vi "APC_9056_TS_loop.vi"(1 "DAQqueue":T3={"Queue array"=[0.0, 0.0, 0.0, 0.0, 0.0, 0.0, 0.0, 0.0, 0.0, 0.0, 0.0, 0.0, 0.0, 0.0, 0.0, 0.0, 0.0, 0.0, 0.0, 0.0, 0.0, 0.0, 0.0, 0.0, 0.0, 0.0, 0.0, 0.0, 0.0, 0.0, 0.0, 0.0, 0.0, 0.0, 0.0, 0.0, 0.0, 0.0, 0.0, 0.0, 0.0, 0.0, 0.0, 0.0, 0.0, 0.0, 0.0, 0.0, 0.0, 0.0, 0.0, 0.0, 0.0, 0.0, 0.0, 0.0, 0.0, 0.0, 0.0, 0.0, 0.0, 0.0, 0.0, 0.0, 0.0, 0.0, 0.0, 0.0, 0.0, 0.0, 0.0], "Channel list"=["TimeStamp9056", "NI9220_0_0", "NI9220_0_1", "NI9220_0_2", "NI9220_0_3", "NI9220_0_4", "NI9220_0_5", "NI9220_0_6", "NI9220_0_7", "NI9220_0_8", "NI9220_0_9", "NI9220_0_10", "NI9220_0_11", "NI9220_0_12", "NI9220_0_13", "NI9220_0_14", "NI9220_0_15", "NI9220_1_0", "NI9220_1_1", "NI9220_1_2", "NI9220_1_3", "NI9220_1_4", "NI9220_1_5", "NI9220_1_6", "NI9220_1_7", "NI9220_1_8", "NI9220_1_9", "NI9220_1_10", "NI9220_1_11", "NI9220_1_12", "NI9220_1_13", "NI9220_1_14", "NI9220_1_15", "Pcyl1", "Pcyl2", "Pcyl3", "Pcyl4", "time_9049_TS", "SystemState", "InjEnable", "MainEnable", "MainDuration", "MainSOI", "SparkEnable", "SparkTiming", "EngineSpeed_rpm", "SystPres", "IMEPg1", "IMEPg2", "IMEPg3", "IMEPg4", "IMEPg5", "IMEPg6", "IMEPn1", "IMEPn2", "IMEPn3", "IMEPn4", "IMEPn5", "IMEPn6", "MaxPcyl1", "MaxPcyl2", "MaxPcyl3", "MaxPcyl4", "MaxPcyl5", "MaxPcyl6", "IMEPstd1", "IMEPstd2", "IMEPstd3", "IMEPstd4", "IMEPstd5", "IMEPstd6"], "TS queue"=refnum, "TS signals path"="/home/lvuser/natinst/LabVIEW Data/APC_10Hz_"}, 2 "error in":errorcluster, 3 "scaled dAQmx task":refnum<k21>[](array[refnum])=["", "", ""]) -> ()   [LabVIEW 2020]
doc: "This example demonstrates the procedure required to apply different NI-DAQmx Custom Scales to each virtual channel in a task. A DAQmx Task Property Node (Functions >> NI Measurements >> DAQmx - Data Acquisition >> DAQmx Advanced Task Options) is used to obtain the task's virtual channels. A DAQmx Channel Property Node (Functions >> NI Measurements >> DAQmx - Data Acquisition) is then used to set the custom scale for each virtual channel in the task.\n\nThe \"DAQmx Create Scale\" VI creates a custom scale for each channel in the channel list. *Note, make sure your Minimum and Maximum channel parameters are consistent with the range the scale will create."
uses:
  controls/APC_ControlSettings.ctl
  controls/APC_PIDcontrolSettings.ctl
  <vilib>/Platform/TimedLoop/XDataNode/timing_clust.ctl
  <vilib>/Platform/TimedLoop/XDataNode/nitl_modes.ctl
  <vilib>/Platform/TimedLoop/XDataNode/wakeup.ctl
  <vilib>/DAQmx/read.llb/DAQmx Read (Analog 2D DBL NChan NSamp).vi
  <vilib>/Analysis/baseanly.llb/Mean (DBL).vi
  <vilib>/DAQmx/miscellaneous.llb/DAQmx Fill In Error Info.vi
  <vilib>/FPGAPlugInAG/cRIO-9056/niLvFpga_Open_cRIO-9056.vi
  <vilib>/rvi/interface/common/dynamic/niFpgaDynamicAddResources.vi
  <vilib>/Utility/error.llb/Error Cluster From Error Code.vi
  <vilib>/rvi/errors/niLvFpgaAdjustHostInterfaceError.vi
  <vilib>/Platform/TimedLoop/XDataNode/XDataNode.xnode
  <vilib>/rvi/interface/nirviOpenFPGA/nirviOpenFPGA.xnode
  FPGA Bitfiles/monarch_FPGATarget2_APC9056FPGAmain_1JKoecJL0LU.lvbitx
  APC_9056_FPGA_main.vi
  <vilib>/rvi/interface/nirviReadWriteControl/nirviReadWriteControl.xnode
  <vilib>/Platform/TimedLoop/XDataNode/XDNodeRunTimeDep.lvlib
  <vilib>/Analysis/NI_AALBase.lvlib
  <resource>/objmgr/daqmx.rc
  NiFpgaLv.dll
  <vilib>/rvi/interface/Simulation/niFpgaSimulationCallBeginRW.vi
  FPGA Bitfiles/monarch_FPGATarget3_APC9053FPGAmain_w2oHWSMkDKM.lvbitx
  APC_9053_FPGA_main.vi
panel:
  out "error out TEST":errorcluster
  out "task out_TEST":refnum<k21>
  out "NumChans_TEST":u32
  out "s? t:f":i8
  out "MTRnotResponding":bool
  out "PCnotResponding":bool
  out "9049notResponding":bool
  out "9056notResponding":bool
  out "PC_ControlSettings":T1={"Spark advance [CADBTDC]"=0.0, "Pref"=0.0, "O2ref"=0.0, "DI advance [CADBTDC]"=0.0, "DI duration [ms] "=0.0, "CO2ref"=0.0, "PFI duration [ms]"=0.0, "IMEP ref"=0.0, "Speed ref"=0.0, "IGN enable"=TRUE, "DI enable"=TRUE, "CL PFI\n lambda"=TRUE, "CL PFI\nIMEP"=FALSE, "Activate\ncylinder"=[FALSE, FALSE, FALSE, FALSE, FALSE, FALSE], "Force idling"=FALSE, "Force motoring"=FALSE, "ETP resync"=FALSE, "Requested mode"=0, "Clear Sync Errors"=FALSE, "toggle TDC"=FALSE, "l ref"=0.0, "PID control references"={"NG"=FALSE, "Ar"=FALSE, "O2"=FALSE, "Intake vent"=FALSE, "Cross vent"=FALSE, "Exhaust vent"=FALSE, "NG control mode"=0, "NG-FC-001-REF"=0.0, "WF-OA-002-REF"=0.0, "IMEP-REF"=0.0, "Nm-REF"=0.0, "Ar control mode"=0, "AR-PC-002-REF"=0.0, "WF-PT-004-REF"=0.0, "O2 control mode"=0, "O2-FC-001-REF"=0.0, "WF-OA-001-REF"=0.0, "Tcoolant control  mode"=0, "EC-FC-001-REF"=0.0, "EC-TT-001-REF"=0.0, "Texh control mode"=0, "SW-FC-004-REF"=0.0, "SW-FT-002-REF"=0.0, "WF-TT-004-REF"=0.0, "Toil control mode"=0, "SW-FC-009-REF"=0.0, "SW-FT-004-REF"=0.0, "EO-TT-001-REF"=0.0, "AIC201_CO2_ConcTarget"=0.0, "O2_FF_NG"=FALSE, "Dyno control mode"=0, "Membrane control mode"=0, "AR-FT-001-REF"=0.0, "MTR modbus floats"=[0.0, 0.0, 0.0, 0.0, 0.0, 0.0, 0.0, 0.0, 0.0, 0.0, 0.0, 0.0, 0.0, 0.0, 0.0, 0.0, 0.0, 0.0, 0.0], "MTR modbus u16"=[0, 0, 0, 0, 0, 0, 0], "MTR HB"=FALSE, "PC_HB"=FALSE, "EMERGENCY STOP"=FALSE}, "CA50setpoint [CADATDC]"=0.0, "CA50 control"=TRUE, "Knock control"=TRUE, "CLEAR EMERGENCY STOP"=FALSE, "EMERGENCY STOP"=FALSE}
  out "error out 2":errorcluster
  out "error out":errorcluster
  out "Channel list":string[](array[string])
  in  "Max file size (MiB)":dbl=150.0
  out "TDMS file size (in bytes)":i64
  in  "Override controllers":bool
  in  "DYNO-REF":dbl
  in  "SW-FC-009-REF":dbl
  in  "SW-FC-004-REF":dbl
  in  "EC-FC-001-REF":dbl
  in  "NG-FC-001-REF":dbl
  in  "AR-PC-002-REF":dbl
  in  "O2-FC-001-REF":dbl
  in  "NI9269/AO3":fxp<+/-,20,5>
  in  "NI9269/AO2":fxp<+/-,20,5>
  in  "NI9269/AO1":fxp<+/-,20,5>
  in  "NI9269/AO0":fxp<+/-,20,5>
  in  "NI9214  (manual)":dbl[](array[numeric])=[0.0, 0.0, 0.0, 0.0, 0.0, 0.0, 0.0, 0.0, 0.0, 0.0, 0.0, 0.0, 0.0, 0.0, 0.0, 0.0, 0.0, 0.0, 0.0, 0.0, 0.0, 0.0, 0.0, 0.0, 0.0, 0.0, 0.0, 0.0, 0.0, 0.0, 0.0, 0.0] format="%0.5f"
  in  "NI9208  (manual)":dbl[](array[numeric])=[-0.0033997970000000004, 4.9987908475000005, 9.990422618, 14.998184486000001, 20.01738117, 25.004057022, 29.988959596500003, 34.99554141, -7.563000000000014e-05, 0.0006727460000000001, -0.0045439285, -0.007908694, -0.0070815059999999996, -0.00245116, 0.008481419, -0.011168849500000001] format="%0.5f"
  in  "ManualState":i8
  in  "ForceState":bool
  in  "emulate 9205":bool
  in  "NI9205  (manual)":dbl[](array[numeric])=[-0.0033997970000000004, 4.9987908475000005, 9.990422618, 14.998184486000001, 20.01738117, 25.004057022, 29.988959596500003, 34.99554141, -7.563000000000014e-05, 0.0006727460000000001, -0.0045439285, -0.007908694, -0.0070815059999999996, -0.00245116, 0.008481419, -0.011168849500000001] format="%0.5f"
  in  "emulate 9214":bool
  in  "emulate 9208":bool
  in  "ExhVent":bool
  in  "CrossVent":bool
  in  "IntVent":bool
  in  "O2":bool
  in  "Ar":bool
  in  "NG":bool
  in  "Override switchs from PC":bool
  out "WF-FC-003":bool
  out "WF-FC-002":bool
  out "WF-FC-001":bool
  out "AR-PV-004":bool
  out "O2-PV-004":bool
  out "NG-FV-001":bool
  out "DYNO-REF":dbl format="%.2f"
  out "AR-PC-002-REF":dbl format="%.2f"
  out "O2-FC-001-REF":dbl format="%.2f"
  out "SW-FC-009-REF":dbl format="%.2f"
  out "EC-FC-001-REF":dbl format="%.2f"
  out "NG-FC-001-REF":dbl format="%.2f"
  out "size(s) 2":i32
  out "SW-FC-004-REF":dbl format="%.2f"
  out "SYSTEM STATE":i8
  out "path":path=path "/home/lvuser/natinst/LabVIEW Data/APC_10Hz_231109_111212_10Hz.tdms"
  out "error out 3":errorcluster
  out "9049_CycleAveragedVariables":dbl[](array[numeric])=[969029.0, 0.0, 0.0, 1.0, 0.0, 0.0, 0.0, 0.0, 1145.6240234375, 0.17644237731943965, 6.8272752501669425, 6.8272752501669425, 6.8272752501669425, 6.8272752501669425, 6.8272752501669425, 6.8272752501669425, 7.153851381122263, 7.153851381122263, 7.153851381122263, 7.153851381122263, 7.153851381122263, 7.153851381122263, 2.315526348, 5.034533782, 14.60978205, 477.4405173, 0.338477399, 0.460883882, 0.0, 0.0, 0.0, 0.0, 0.0, 0.0]
  out "elapsed time 9205":u32=100
  out "elapsed time 9208":u32=100
  out "elapsed time 9214":u32=99
  out "AODODI_raster":dbl[](array[numeric])
  in  "NI9375/DO15":bool
  in  "NI9375/DO14":bool
  in  "NI9375/DO13":bool
  in  "NI9375/DO12":bool
  in  "NI9375/DO11":bool
  in  "NI9375/DO10":bool
  in  "NI9375/DO9":bool
  in  "NI9375/DO8":bool
  in  "NI9375/DO7":bool
  in  "NI9375/DO6":bool
  out "NI9375/DO5":bool
  out "NI9375/DO4":bool
  out "NI9375/DO3":bool
  out "NI9375/DO2":bool
  out "NI9375/DO1":bool
  out "NI9375/DO0":bool
  in  "NI9266/AO7":fxp<+,20,-5>
  out "NI9266/AO6":fxp<+,20,-5>
  out "NI9266/AO5":fxp<+,20,-5>
  out "NI9266/AO4":fxp<+,20,-5>
  out "NI9266/AO3":fxp<+,20,-5>
  out "NI9266/AO2":fxp<+,20,-5>
  out "NI9266/AO1":fxp<+,20,-5>
  out "NI9266/AO0":fxp<+,20,-5>
  out "NI9375/DI15":bool
  out "NI9375/DI14":bool
  out "NI9375/DI13":bool
  out "NI9375/DI12":bool
  out "NI9375/DI11":bool
  out "NI9375/DI10":bool
  out "NI9375/DI9":bool
  out "NI9375/DI8":bool
  out "NI9375/DI7":bool
  out "NI9375/DI6":bool
  out "NI9375/DI5":bool
  out "NI9375/DI4":bool
  out "NI9375/DI3":bool
  out "NI9375/DI2":bool
  out "NI9375/DI1":bool
  out "NI9375/DI0":bool
  in  "NI9264/AO15":fxp<+/-,20,5>
  in  "NI9264/AO14":fxp<+/-,20,5>
  in  "NI9264/AO13":fxp<+/-,20,5>
  in  "NI9264/AO12":fxp<+/-,20,5>
  in  "NI9264/AO11":fxp<+/-,20,5>
  in  "NI9264/AO10":fxp<+/-,20,5>
  in  "NI9264/AO9":fxp<+/-,20,5>
  in  "NI9264/AO8":fxp<+/-,20,5>
  in  "NI9264/AO7":fxp<+/-,20,5>
  in  "NI9264/AO6":fxp<+/-,20,5>
  in  "NI9264/AO5":fxp<+/-,20,5>
  in  "NI9264/AO4":fxp<+/-,20,5>
  in  "NI9264/AO3":fxp<+/-,20,5>
  in  "NI9264/AO2":fxp<+/-,20,5>
  in  "NI9264/AO1":fxp<+/-,20,5>
  in  "NI9264/AO0":fxp<+/-,20,5>
  out "NI9214":dbl[](array[numeric])=[0.0010449026000000034, 4.999450598799999, 10.0006558688, 14.981061165000003] format="%0.2f"
  out "NI9208":dbl[](array[numeric])=[-0.0033997970000000004, 4.9987908475000005, 9.990422618, 14.998184486000001, 20.01738117, 25.004057022, 29.988959596500003, 34.99554141, -7.563000000000014e-05, 0.0006727460000000001, -0.0045439285, -0.007908694, -0.0070815059999999996, -0.00245116, 0.008481419, -0.011168849500000001] format="%0.5f"
  out "NI9205":dbl[](array[numeric])=[-0.00361437722, 5.001652418760002, 9.99553711734999, 14.990208086199992, 19.993287157860003, 24.99203765954996, 29.986607142530012, 34.99718714015995, -0.001139086, -0.009304434079999986, -2.86875499999999e-05, 0.003279013959999996, -0.0027344005399999993, -0.0021136663599999996, -6.22128e-05, -0.006222946800000002] format="%0.2f"
  # "With the current number of channels 159 MiB is equal to 2 h of recording. The system creates a new file if the file size is exceeded. The size limit is for avoiding huge files difficult to open."
  # "APC_9056_WatchDog Output"
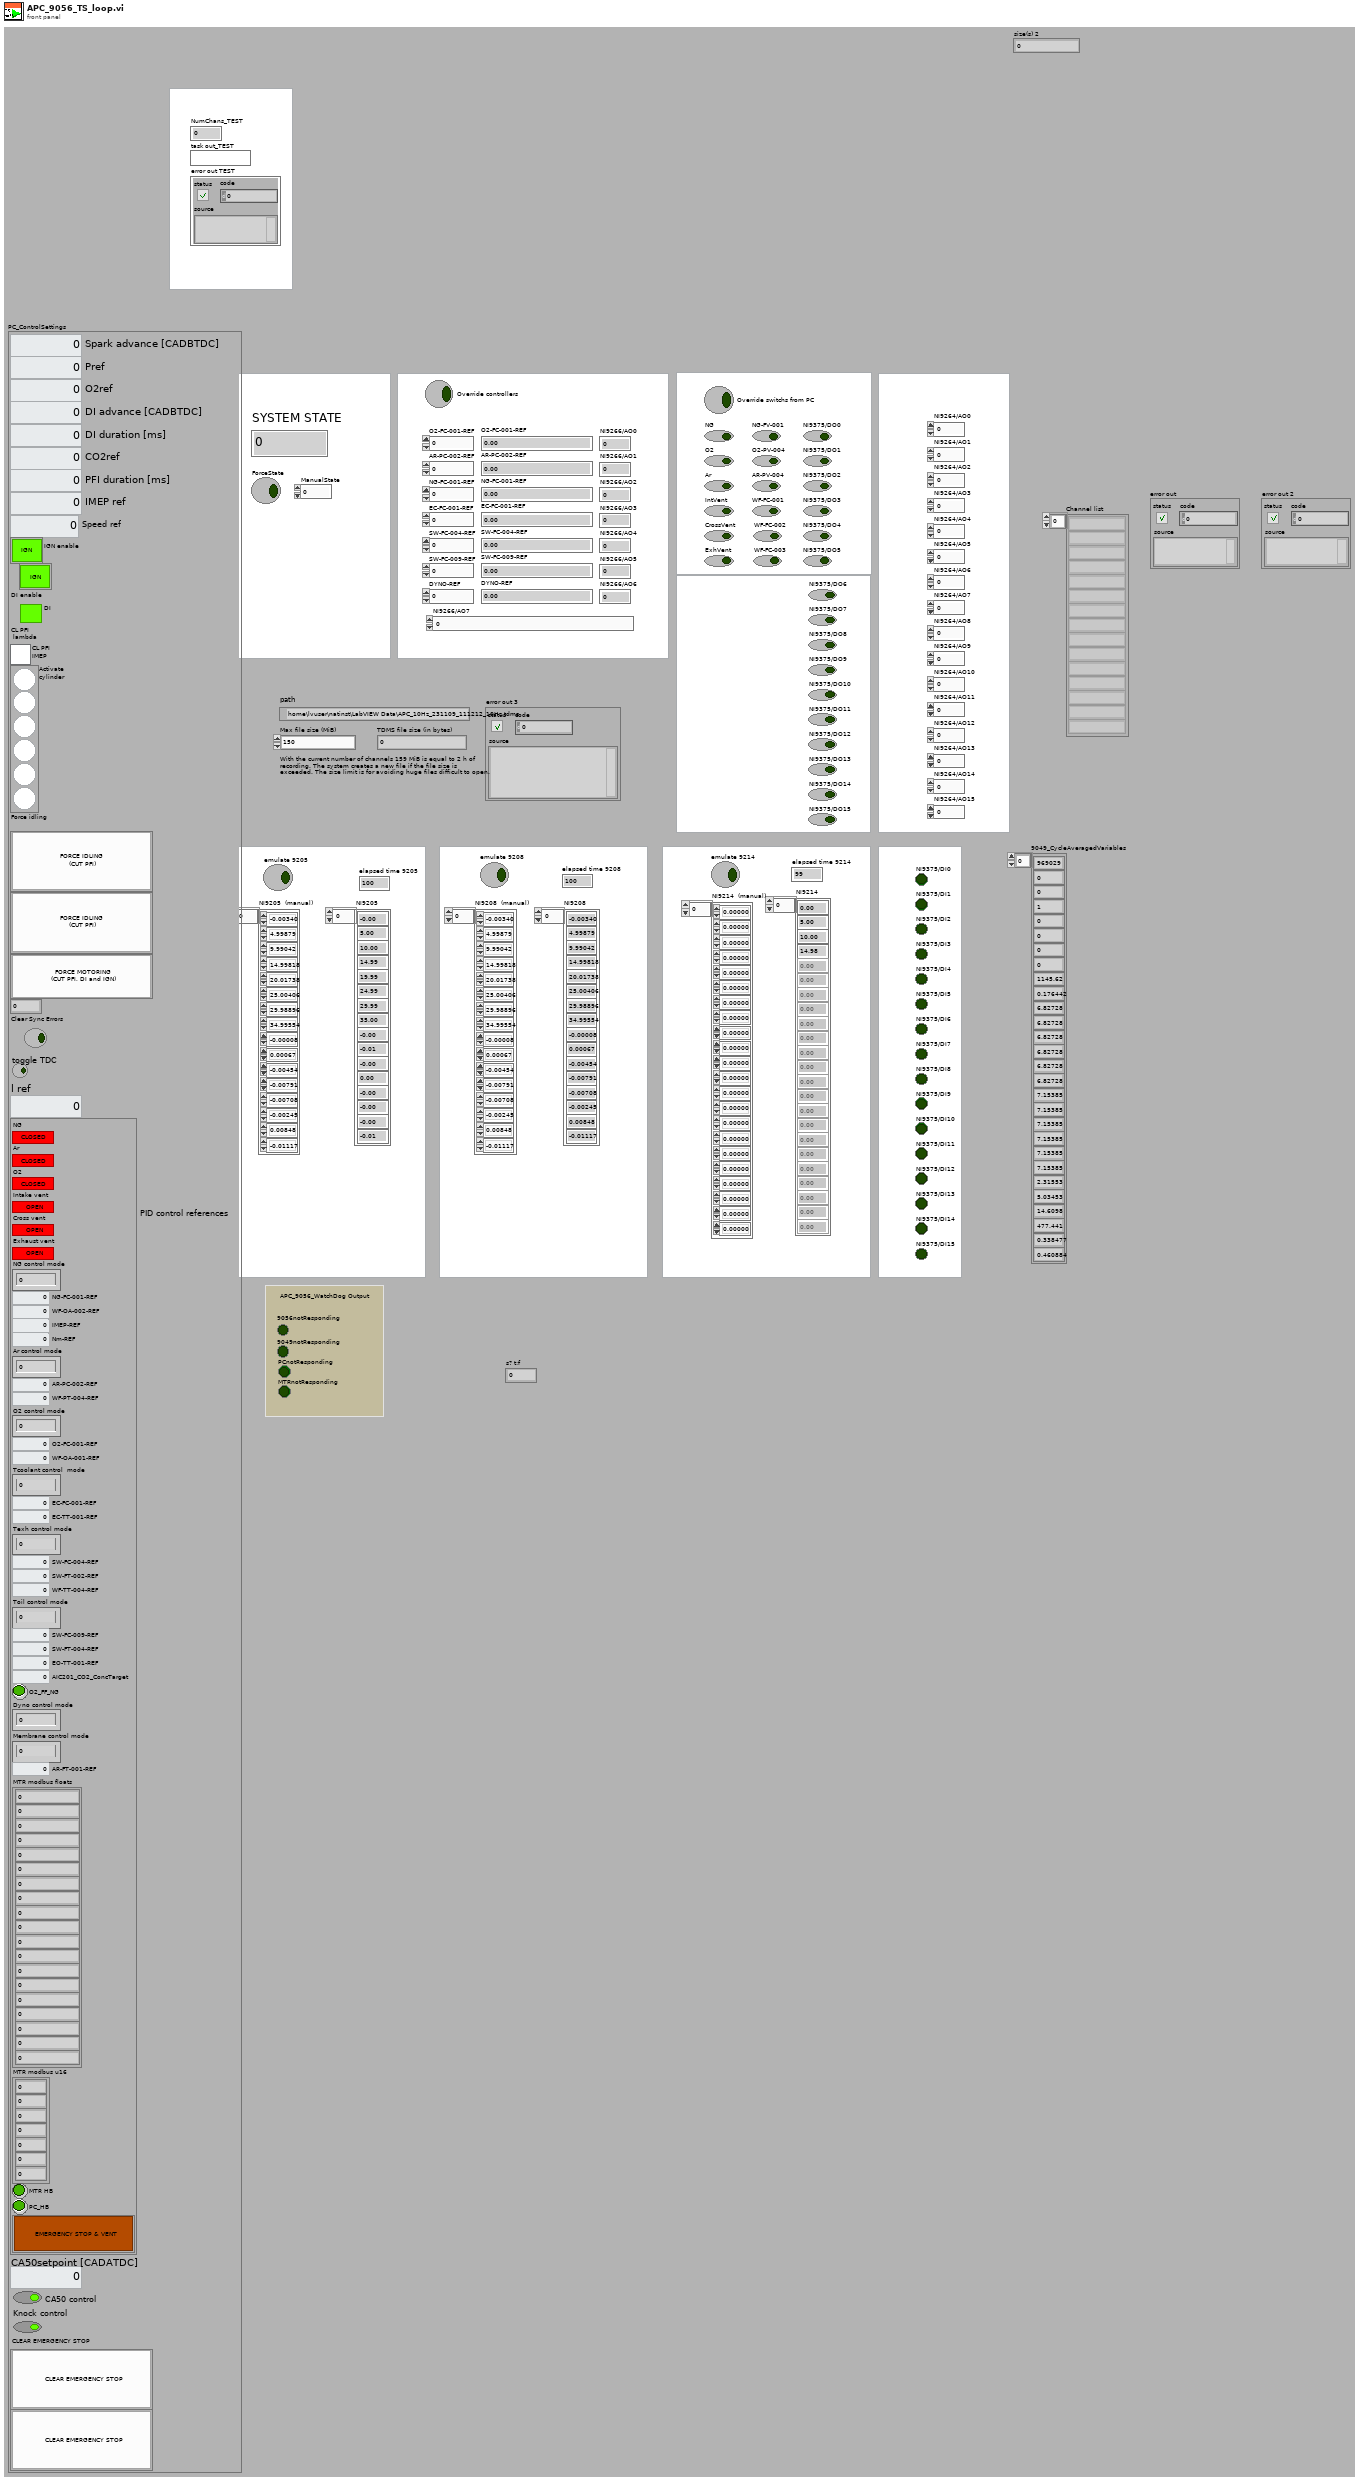
[diagram p1: front panel]
types:
  T1 = typedef "APC_ControlSettings.ctl" = cluster{"Spark advance [CADBTDC]":dbl, "Pref":dbl, "O2ref":dbl, "DI advance [CADBTDC]":dbl, "DI duration [ms] ":dbl, "CO2ref":dbl, "PFI duration [ms]":dbl, "IMEP ref":dbl, "Speed ref":dbl, "IGN enable":bool, "DI enable":bool, "CL PFI\n lambda":bool, "CL PFI\nIMEP":bool, "Activate\ncylinder":bool[], "Force idling":bool, "Force motoring":bool, "ETP resync":bool, "Requested mode":i8, "Clear Sync Errors":bool, "toggle TDC":bool, "l ref":dbl, "PID control references":T2, "CA50setpoint [CADATDC]":dbl, "CA50 control":bool, "Knock control":bool, "CLEAR EMERGENCY STOP":bool, "EMERGENCY STOP":bool}
  T2 = typedef "APC_PIDcontrolSettings.ctl" = cluster{"NG":bool, "Ar":bool, "O2":bool, "Intake vent":bool, "Cross vent":bool, "Exhaust vent":bool, "NG control mode":u8, "NG-FC-001-REF":dbl, "WF-OA-002-REF":dbl, "IMEP-REF":dbl, "Nm-REF":dbl, "Ar control mode":u8, "AR-PC-002-REF":dbl, "WF-PT-004-REF":dbl, "O2 control mode":u8, "O2-FC-001-REF":dbl, "WF-OA-001-REF":dbl, "Tcoolant control  mode":u8, "EC-FC-001-REF":dbl, "EC-TT-001-REF":dbl, "Texh control mode":u8, "SW-FC-004-REF":dbl, "SW-FT-002-REF":dbl, "WF-TT-004-REF":dbl, "Toil control mode":u8, "SW-FC-009-REF":dbl, "SW-FT-004-REF":dbl, "EO-TT-001-REF":dbl, "AIC201_CO2_ConcTarget":dbl, "O2_FF_NG":bool, "Dyno control mode":u8, "Membrane control mode":u8, "AR-FT-001-REF":dbl, "MTR modbus floats":sgl[], "MTR modbus u16":u16[], "MTR HB":bool, "PC_HB":bool, "EMERGENCY STOP":bool}
  T3 = cluster{"Queue array":dbl[], "Channel list":string[], "TS queue":refnum<queue>, "TS signals path":string}
  T4 = typedef "XDNodeRunTimeDep.lvlib/timing_clust.ctl" = cluster{"Expected End [f-1]":u64, "Actual End [f-1]":u64, "Finished Late? [f-1]":bool, "Expected End [i-1]":u64, "Actual End [i-1]":u64, "Finished Late? [i-1]":bool, "Expected Start [i]":u64, "Actual Start [i]":u64, "Expected Start [f]":u64, "Actual Start [f]":u64, "Source Name":string, "Structure Name":string, "Period":i64, "Deadline":i64, "Offset":i64, "Start":i64, "Priority":i32, "Timeout":i32, "Mode":T5, "Wakeup Reason":T6, "Error":errorcluster, "Source Type":string, "Secondary Source Type":string, "Global End Time":u64, "Global Start Time":u64, "Frame Duration":u64, "Iteration Duration":u64, "Assigned CPU":i32, "I/O Scan Engine Mode":u32}
  T5 = typedef "XDNodeRunTimeDep.lvlib/nitl_modes.ctl" = enum32{"No Change", "Process missed periods, maintain original phase", "Discard missed periods, maintain original phase", "Process missed periods, ignore original phase", "Discard missed periods, ignore original phase"}
  T6 = typedef "XDNodeRunTimeDep.lvlib/wakeup.ctl" = enum32{"Normal", "Aborted", "Asynchronous wakeup", "Timing source error", "Timed loop error", "Timeout"}
  T7 = enum16{"open", "open or create", "create or replace", "create", "open (read-only)"}
  T8 = typedef "APC_PIDCluster.ctl" = cluster{"AR-FT-001":dbl, "O2-FC-001":dbl, "SW-FT-004":dbl, "SW-FT-002":dbl, "WF-OA-002":dbl, "WF-PT-004":dbl, "WF-OA-001":dbl, "EC-TT-001":dbl, "WF-TT-004":dbl, "EC-FC-001":dbl, "NG-FC-001":dbl, "EO-TT-001":dbl, "SW-FC-008":dbl, "SW-FC-004":dbl, "IMEPn6":dbl, "TORQUE":dbl, "CylPresWarnings":dbl, "CylPresErrors":dbl, "NG-FT-001":dbl, "EngineSpeed_rpm":dbl}
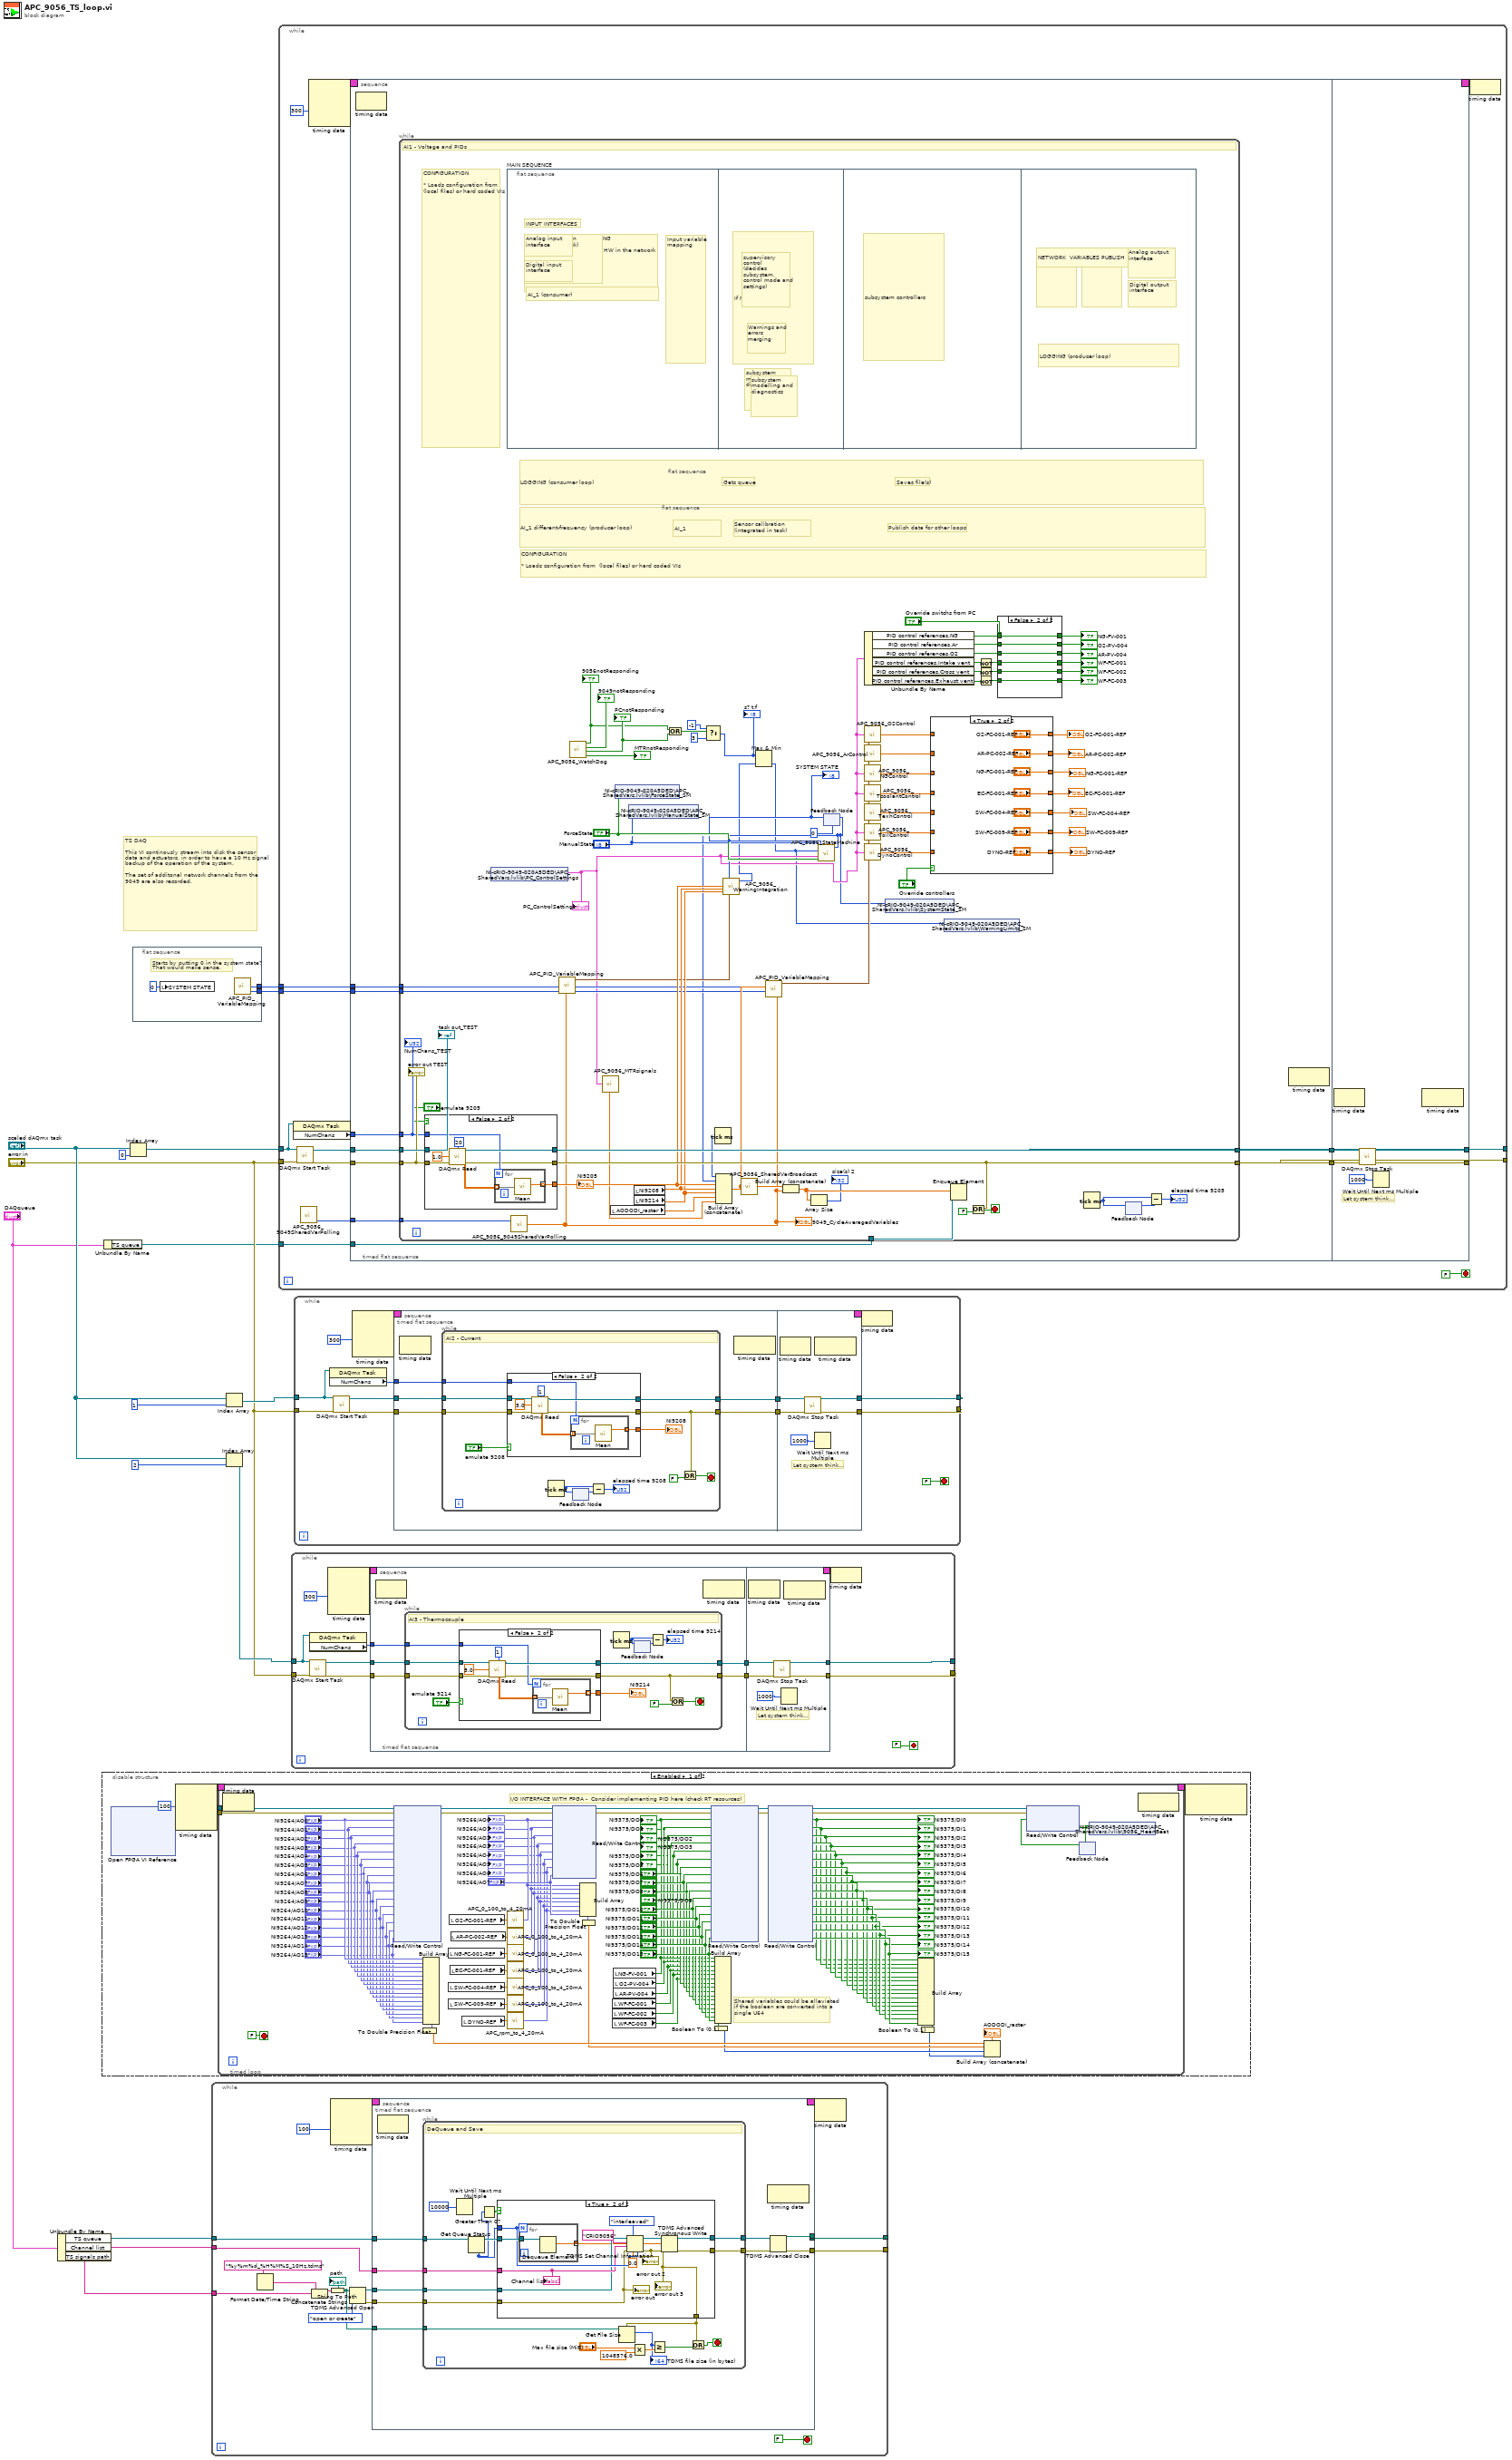
[diagram p0: block diagram]
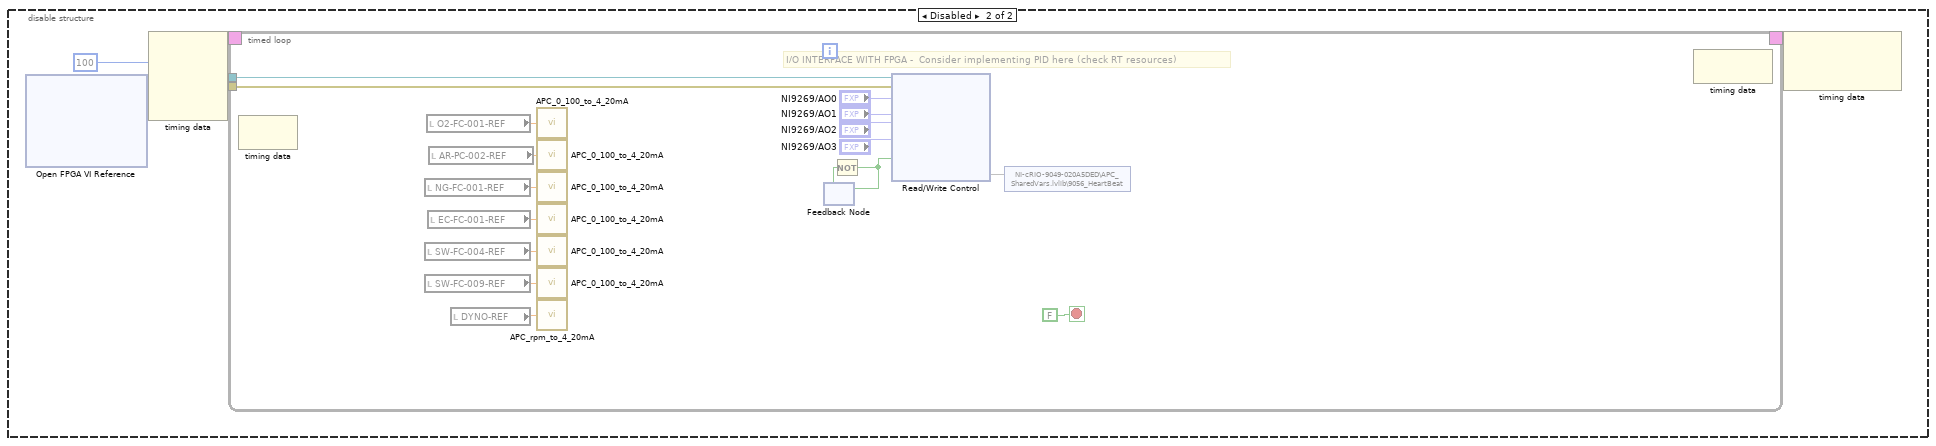
[diagram p2: hidden frame]
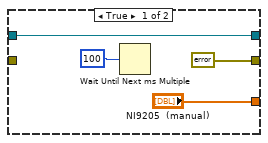
[diagram p5: hidden frame]
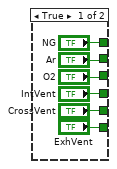
[diagram p6: hidden frame]
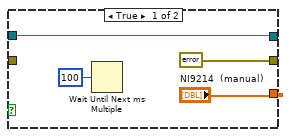
[diagram p7: hidden frame]
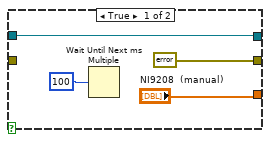
[diagram p8: hidden frame]
diagram:
  # "TS DAQ\n\nThis VI continously stream into disk the sensor data and actuators, in order to have a 10 Hz signal backup of the operation of the system.\n\nThe set of additonal network channels from the 9049 are also recorded."
  n1 = Unbundle By Name("DAQqueue") -> ("TS queue"=w13:refnum<queue>, "Channel list"=w11:string[], "TS signals path"=w10:string)
  n2 = disable-structure shown="Enabled" {
    frame Enabled {
      n3 = xnode "Open FPGA VI Reference"() -> ("FPGA VI Reference Out"=w18:refnum<k20>, "error out"=w17:errorcluster)  [unwired: 2 in]
      n4 = node-c288(i64 100 ("Period")) -> (w20:T4)  [unwired: 3 in]
      n5 = timed-loop {
        tunnel: w18 -> [w101]
        tunnel: w17 -> [w100]
        timing: w20 -> [_]
        timing-out: [_] -> w19
        stop <- FALSE ("Stop DAQ 7") stop-if-true
        # "Shared variables could be alleviated if the boolean are converted into a single U64"
        # "I/O INTERFACE WITH FPGA -  Consider implementing PID here (check RT resources)"
        n6 = node-c288() -> ()  [unwired: 1 in, 1 out]
        n7 = xnode "Read/Write Control"("FPGA VI Reference In"=w101, "error in"=w100, "NI9264/AO0"="NI9264/AO0", "NI9264/AO1"="NI9264/AO1", "NI9264/AO2"="NI9264/AO2", "NI9264/AO3"="NI9264/AO3", "NI9264/AO4"="NI9264/AO4", "NI9264/AO5"="NI9264/AO5", "NI9264/AO6"="NI9264/AO6", "NI9264/AO7"="NI9264/AO7", "NI9264/AO8"="NI9264/AO8", "NI9264/AO9"="NI9264/AO9", "NI9264/AO10"="NI9264/AO10", "NI9264/AO11"="NI9264/AO11", "NI9264/AO12"="NI9264/AO12", "NI9264/AO13"="NI9264/AO13", "NI9264/AO14"="NI9264/AO14", "NI9264/AO15"="NI9264/AO15") -> ("FPGA VI Reference Out"=w104:refnum<k20>, "error out"=w99:errorcluster)
        n8 = Build Array("NI9264/AO0", "NI9264/AO1", "NI9264/AO2", "NI9264/AO3", "NI9264/AO4", "NI9264/AO5", "NI9264/AO6", "NI9264/AO7", "NI9264/AO8", "NI9264/AO9", "NI9264/AO10", "NI9264/AO11", "NI9264/AO12", "NI9264/AO13", "NI9264/AO14", "NI9264/AO15") -> (w79:fxp<+/-,20,5>[])
        n9 = To Double Precision Float(number=w79) -> (double precision float=w50:dbl[])
        n10 = local read "NG-FC-001-REF"() -> (w40:dbl)
        n11 = local read "SW-FC-004-REF"() -> (w38:dbl)
        n12 = local read "SW-FC-009-REF"() -> (w37:dbl)
        n13 = local read "O2-FC-001-REF"() -> (w42:dbl)
        n14 = local read "EC-FC-001-REF"() -> (w39:dbl)
        n15 = local read "AR-PC-002-REF"() -> (w41:dbl)
        n16 = local read "DYNO-REF"() -> (w36:dbl)
        n17 = call "APC_0_100_to_4_20mA.vi"("Perc0_100"=w42) -> ("fixed-point"=w35:fxp<+,20,-5>)
        "NI9266/AO0" <- w35
        n18 = call "APC_0_100_to_4_20mA.vi"("Perc0_100"=w41) -> ("fixed-point"=w34:fxp<+,20,-5>)
        "NI9266/AO1" <- w34
        n19 = call "APC_0_100_to_4_20mA.vi"("Perc0_100"=w40) -> ("fixed-point"=w33:fxp<+,20,-5>)
        "NI9266/AO2" <- w33
        n20 = call "APC_0_100_to_4_20mA.vi"("Perc0_100"=w39) -> ("fixed-point"=w32:fxp<+,20,-5>)
        "NI9266/AO3" <- w32
        n21 = call "APC_0_100_to_4_20mA.vi"("Perc0_100"=w38) -> ("fixed-point"=w31:fxp<+,20,-5>)
        "NI9266/AO4" <- w31
        n22 = call "APC_0_100_to_4_20mA.vi"("Perc0_100"=w37) -> ("fixed-point"=w30:fxp<+,20,-5>)
        "NI9266/AO5" <- w30
        n23 = call "APC_rpm_to_4_20mA.vi"("Perc0_100"=w36) -> ("fixed-point"=w29:fxp<+,20,-5>)
        "NI9266/AO6" <- w29
        n24 = xnode "Read/Write Control"("FPGA VI Reference In"=w104, "error in"=w99, "NI9266/AO0"=w35, "NI9266/AO1"=w34, "NI9266/AO2"=w33, "NI9266/AO3"=w32, "NI9266/AO4"=w31, "NI9266/AO5"=w30, "NI9266/AO6"=w29, "NI9266/AO7"="NI9266/AO7") -> ("FPGA VI Reference Out"=w103:refnum<k20>, "error out"=w98:errorcluster)
        n25 = Build Array(w35, w34, w33, w32, w31, w30, w29, "NI9266/AO7") -> (w78:fxp<+,20,-5>[])
        n26 = To Double Precision Float(number=w78) -> (double precision float=w49:dbl[])
        n27 = local read "WF-FC-001"() -> (w25:bool)
        "NI9375/DO3" <- w25
        n28 = local read "WF-FC-002"() -> (w24:bool)
        "NI9375/DO4" <- w24
        n29 = local read "WF-FC-003"() -> (w23:bool)
        "NI9375/DO5" <- w23
        n30 = local read "NG-FV-001"() -> (w28:bool)
        "NI9375/DO0" <- w28
        n31 = local read "O2-PV-004"() -> (w27:bool)
        "NI9375/DO1" <- w27
        n32 = local read "AR-PV-004"() -> (w26:bool)
        "NI9375/DO2" <- w26
        n33 = xnode "Read/Write Control"("FPGA VI Reference In"=w103, "error in"=w98, "NI9375/DO0"=w28, "NI9375/DO1"=w27, "NI9375/DO2"=w26, "NI9375/DO3"=w25, "NI9375/DO4"=w24, "NI9375/DO5"=w23, "NI9375/DO6"="NI9375/DO6", "NI9375/DO7"="NI9375/DO7", "NI9375/DO8"="NI9375/DO8", "NI9375/DO9"="NI9375/DO9", "NI9375/DO10"="NI9375/DO10", "NI9375/DO11"="NI9375/DO11", "NI9375/DO12"="NI9375/DO12", "NI9375/DO13"="NI9375/DO13", "NI9375/DO14"="NI9375/DO14", "NI9375/DO15"="NI9375/DO15") -> ("FPGA VI Reference Out"=w102:refnum<k20>, "error out"=w97:errorcluster)
        n34 = Build Array(w28, w27, w26, w25, w24, w23, "NI9375/DO6", "NI9375/DO7", "NI9375/DO8", "NI9375/DO9", "NI9375/DO10", "NI9375/DO11", "NI9375/DO12", "NI9375/DO13", "NI9375/DO14", "NI9375/DO15") -> (w45:bool[])
        n35 = Boolean To (0,1)(Boolean=w45) -> (0, 1=w48:i16[])
        n36 = xnode "Read/Write Control"("FPGA VI Reference In"=w102, "error in"=w97) -> ("FPGA VI Reference Out"=w44:refnum<k20>, "error out"=w43:errorcluster, "NI9375/DI0"=w51:bool, "NI9375/DI1"=w52:bool, "NI9375/DI2"=w53:bool, "NI9375/DI3"=w54:bool, "NI9375/DI4"=w55:bool, "NI9375/DI5"=w56:bool, "NI9375/DI6"=w57:bool, "NI9375/DI7"=w58:bool, "NI9375/DI8"=w59:bool, "NI9375/DI9"=w60:bool, "NI9375/DI10"=w61:bool, "NI9375/DI11"=w62:bool, "NI9375/DI12"=w63:bool, "NI9375/DI13"=w64:bool, "NI9375/DI14"=w65:bool, "NI9375/DI15"=w66:bool)
        "NI9375/DI0" <- w51
        "NI9375/DI1" <- w52
        "NI9375/DI2" <- w53
        "NI9375/DI3" <- w54
        "NI9375/DI4" <- w55
        "NI9375/DI5" <- w56
        "NI9375/DI6" <- w57
        "NI9375/DI7" <- w58
        "NI9375/DI8" <- w59
        "NI9375/DI9" <- w60
        "NI9375/DI10" <- w61
        "NI9375/DI11" <- w62
        "NI9375/DI12" <- w63
        "NI9375/DI13" <- w64
        "NI9375/DI14" <- w65
        "NI9375/DI15" <- w66
        n37 = Build Array(w51, w52, w53, w54, w55, w56, w57, w58, w59, w60, w61, w62, w63, w64, w65, w66) -> (w67:bool[])
        n38 = Boolean To (0,1)(Boolean=w67) -> (0, 1=w47:i16[])
        n39 = Build Array (concatenate)(w50, w49, w48, w47) -> (→"AODODI_raster":dbl[])
        n40 = feedback #1() -> (w22:bool)  [unwired: 1 in]
        n41 = xnode "Read/Write Control"("FPGA VI Reference In"=w44, "error in"=w43, "RT watchdog"=w22) -> ("FPGA Hearbeat"=w21:bool)  [unwired: 2 out]
        n42 = feedback-in #1(w21) -> ()
        n43 = shared-variable "NI-cRIO-9049-020A5DED\\APC_SharedVars.lvlib\\9056_HeartBeat"(w21) -> ()  [unwired: 1 in, 1 out]
        n44 = node-c288() -> ()  [unwired: 1 in, 1 out]
      }
      n45 = node-c288(w19) -> ()  [unwired: 2 out]
    }
    frame Disabled {
      n46 = xnode "Open FPGA VI Reference"() -> ("FPGA VI Reference Out"=w114:refnum<k20>, "error out"=w113:errorcluster)  [unwired: 2 in]
      n47 = node-c288(i64 100 ("Period")) -> (w116:T4)  [unwired: 3 in]
      n48 = timed-loop {
        tunnel: w114 -> [w132]
        tunnel: w113 -> [w131]
        timing: w116 -> [_]
        timing-out: [_] -> w115
        stop <- FALSE ("Stop DAQ 8") stop-if-true
        # "I/O INTERFACE WITH FPGA -  Consider implementing PID here (check RT resources)"
        n49 = node-c288() -> ()  [unwired: 1 in, 1 out]
        n50 = local read "NG-FC-001-REF"() -> (w125:dbl)
        n51 = local read "SW-FC-004-REF"() -> (w123:dbl)
        n52 = local read "SW-FC-009-REF"() -> (w122:dbl)
        n53 = local read "O2-FC-001-REF"() -> (w127:dbl)
        n54 = local read "EC-FC-001-REF"() -> (w124:dbl)
        n55 = local read "AR-PC-002-REF"() -> (w126:dbl)
        n56 = local read "DYNO-REF"() -> (w121:dbl)
        n57 = call "APC_0_100_to_4_20mA.vi"("Perc0_100"=w127) -> ()  [unwired: 1 out]
        n58 = call "APC_0_100_to_4_20mA.vi"("Perc0_100"=w126) -> ()  [unwired: 1 out]
        n59 = call "APC_0_100_to_4_20mA.vi"("Perc0_100"=w125) -> ()  [unwired: 1 out]
        n60 = call "APC_0_100_to_4_20mA.vi"("Perc0_100"=w124) -> ()  [unwired: 1 out]
        n61 = call "APC_0_100_to_4_20mA.vi"("Perc0_100"=w123) -> ()  [unwired: 1 out]
        n62 = call "APC_0_100_to_4_20mA.vi"("Perc0_100"=w122) -> ()  [unwired: 1 out]
        n63 = call "APC_rpm_to_4_20mA.vi"("Perc0_100"=w121) -> ()  [unwired: 1 out]
        n64 = feedback #2() -> (w129:bool)  [unwired: 1 in]
        n65 = Not(x=w129) -> (.not. x?=w130:bool)
        n66 = feedback-in #2(w130) -> ()
        n67 = xnode "Read/Write Control"("FPGA VI Reference In"=w132, "error in"=w131, "NI9269/AO0"="NI9269/AO0", "NI9269/AO1"="NI9269/AO1", "NI9269/AO2"="NI9269/AO2", "NI9269/AO3"="NI9269/AO3", "RT watchdog"=w130) -> ("FPGA Hearbeat"=w128)  [unwired: 2 out]
        n68 = shared-variable "NI-cRIO-9049-020A5DED\\APC_SharedVars.lvlib\\9056_HeartBeat"(w128) -> ()  [unwired: 1 in, 1 out]
        n69 = node-c288() -> ()  [unwired: 1 in, 1 out]
      }
      n70 = node-c288(w115) -> ()  [unwired: 2 out]
    }
  }
  n71 = Unbundle By Name("DAQqueue") -> ("TS queue"=w4:refnum<queue>)
  n72 = Index Array(array="scaled dAQmx task", index=0) -> (element=w3:refnum<k21>)
  n73 = flat-sequence {
    tunnel: [w142] -> w2
    tunnel: [w141] -> w1
    frame #0 {
      # "Starts by putting 0 in the system state?\nThat would make sense."
      n74 = local write "SYSTEM STATE"(i8 0 ("SYSTEM STATE")) -> ()
      n75 = call "APC_PID_VariableMapping.vi"() -> ("Index 9056"=w141:i32[], "Index 9049"=w142:i32[])  [unwired: 4 in, 1 out]
    }
  }
  n76 = while {
    tunnel: w13 -> [w155]
    tunnel: w11 -> [w154]
    tunnel: [w152] -> _
    tunnel: [w151] -> _
    tunnel: w10 -> [w145]
    stop <- FALSE ("Stop DAQ 11") stop-if-true
    n77 = Format Date/Time String(time format string (%c)="%y%m%d_%H%M%S_10Hz.tdms") -> (date/time string=w144:string)  [unwired: 2 in]
    n78 = Concatenate Strings(w145, w144) -> (w148:string)
    n79 = String To Path(string=w148) -> (path=w143:path)
    "path" <- w143
    n80 = node-c288(100 ("Priority")) -> (w158:T4)  [unwired: 3 in]
    n81 = TDMS Advanced Open(10:T7."open or create" ("operation (0:open)"), 11:w143) -> (0:w149:errorcluster, 3:w150:refnum<k34>)  [unwired: 3 in, 1 out]
    n82 = timed-sequence {
      timing: w158 -> [_]
      timing-out: [_] -> w157
      tunnel: w155 -> [w165]
      tunnel: w154 -> [w164]
      tunnel: [w163] -> w152
      tunnel: [w162] -> w151
      tunnel: w150 -> [w161]
      tunnel: w149 -> [w160]
      tunnel: w143 -> [w159]
      n83 = timed-flat-sequence {
        tunnel: w165 -> [w174]
        tunnel: w164 -> [w173]
        tunnel: [w172] -> w163
        tunnel: [w171] -> w162
        tunnel: w161 -> [w170]
        tunnel: w160 -> [w169]
        tunnel: w159 -> [w166]
        n84 = node-c288() -> ()  [unwired: 1 in, 1 out]
        n85 = while {
          tunnel: w174 -> [w192]
          tunnel: w173 -> [w190]
          tunnel: w170 -> [w187]
          tunnel: w169 -> [w186]
          tunnel: [w185] -> w168
          tunnel: [w184] -> w167
          tunnel: w166 -> [w183]
          stop <- w178 stop-if-true
          # "DeQueue and Save"
          n86 = Wait Until Next ms Multiple(millisecond multiple=u32 10000 ("milliseconds to wait")) -> ()  [unwired: 1 out]
          n87 = Get Queue Status(queue=w192) -> (queue out=w191:refnum<queue>, # elements in queue=w188:i32)  [unwired: 2 in, 6 out]
          n88 = Greater Than 0?(x=w188) -> (x > 0?=w189:bool)
          n89 = case shown="True" w189 {
            tunnel: w191 -> [_ w208]
            tunnel: w188 -> [_ w206]
            tunnel: w190 -> [_ w203]
            tunnel: [w195 w202] -> w185
            tunnel: [w194 w196] -> w184
            tunnel: w187 -> [w195 w201]
            tunnel: w186 -> [w194 w200]
            tunnel: [w194 w196] -> w176
            frame False {
            }
            frame True {
              n90 = for {
                N: w206 -> [_]
                tunnel: w208 -> [w210]
                tunnel: [w209] -> w198 mode=concatenating
                n91 = Dequeue Element(queue=w210) -> (element=w209:dbl[])  [unwired: 2 in, 3 out]
              }
              n92 = TDMS Set Channel Information(4:w206, 6:0.0 ("data type"), 7:enum16{"non-interleaved", "interleaved"}."interleaved" ("data layout (0:non-interleaved)"), 8:w200, 9:w203, 10:"CRIO9056" ("group name (Untitled)"), 11:w201) -> (0:w204:errorcluster, 3:w205:refnum<k34>)
              "error out 2" <- w204
              n93 = TDMS Advanced Synchronous Write(8:w204, 10:w198, 11:w205) -> (0:w196:errorcluster, 3:w202:refnum<k34>)
              "error out 3" <- w196
              "Channel list" <- w203
              "error out" <- w200
            }
          }
          n94 = Get File Size(file=w183, error in=w176) -> (size (in bytes)=w179:i64)  [unwired: 2 out]
          "TDMS file size (in bytes)" <- w179
          n95 = Multiply(x="Max file size (MiB)", y=1048576.0) -> (x*y=w180:dbl)
          n96 = Greater Or Equal?(x=w179, y=w180) -> (x >= y?=w177:bool)
          n97 = Or(x=w176, y=w177) -> (x .or. y?=w178:bool)
        }
        n98 = node-c288() -> ()  [unwired: 1 in, 1 out]
        n99 = TDMS Advanced Close(8:w167, 11:w168) -> (0:w171:errorcluster, 3:w172:path)  [unwired: 2 in]
      }
    }
    n100 = node-c288(w157) -> ()  [unwired: 1 out]
  }
  n101 = Index Array(array="scaled dAQmx task", index=1) -> (element=w8:refnum<k21>)
  n102 = Index Array(array="scaled dAQmx task", index=2) -> (element=w7:refnum<k21>)
  n103 = while {
    tunnel: w3 -> [w220]
    tunnel: "error in" -> [w227]
    tunnel: [w224] -> _
    tunnel: [w223] -> _
    tunnel: w4 -> [w221]
    tunnel: w2 -> [w217]
    tunnel: w1 -> [w216]
    stop <- FALSE ("Stop DAQ 2") stop-if-true
    n104 = property class="DAQmx Task"(reference=w220) -> ("NumChans"=w219:u32)  [unwired: 1 in, 2 out]
    n105 = call <vilib>:"DAQmx Start Task.vi"("task/channels in"=w220, "error in"=w227) -> ("task out"=w226:refnum<k21>, "error out"=w225:errorcluster)  [unwired: 12 in]
    n106 = call "APC_9056_9049SharedVarPolling.vi"() -> ("Number of signals (out)"=w218:i32)  [unwired: 1 in, 1 out]
    n107 = node-c288(300 ("Priority")) -> (w230:T4)  [unwired: 3 in]
    n108 = timed-sequence {
      timing: w230 -> [_]
      timing-out: [_] -> w229
      tunnel: w226 -> [w241]
      tunnel: w225 -> [w240]
      tunnel: [w237] -> w224
      tunnel: [w236] -> w223
      tunnel: w221 -> [w235]
      tunnel: w219 -> [w234]
      tunnel: w218 -> [w233]
      tunnel: w217 -> [w232]
      tunnel: w216 -> [w231]
      n109 = timed-flat-sequence {
        tunnel: w241 -> [w250]
        tunnel: w240 -> [w249]
        tunnel: [w248] -> w239
        tunnel: [w247] -> w238
        tunnel: w235 -> [w246]
        tunnel: w234 -> [w245]
        tunnel: w233 -> [w244]
        tunnel: w232 -> [w243]
        tunnel: w231 -> [w242]
        tunnel: w239 -> [w372]
        tunnel: w238 -> [w371]
        tunnel: [w370] -> w237
        tunnel: [w369] -> w236
        frame #0 {
          n110 = node-c288() -> ()  [unwired: 1 in, 1 out]
          n111 = while {
            tunnel: w250 -> [w326]
            tunnel: w249 -> [w325]
            tunnel: [w324] -> w248
            tunnel: [w318] -> w247
            tunnel: w246 -> [w323]
            tunnel: w245 -> [w322]
            tunnel: w244 -> [w315]
            tunnel: w243 -> [w285]
            tunnel: w242 -> [w284]
            stop <- w316 stop-if-true
            # "CONFIGURATION\n\n* Loads configuration from  (local files) or hard coded VIs"
            # "CONFIGURATION\n\n* Loads configuration from  (local files) or hard coded VIs"
            # "AI_1 different-frequency (producer loop)"
            # "LOGGING (consumer loop)"
            # "AI1 - Voltage and PIDs"
            n112 = case shown="False" "emulate 9205" {
              tunnel: w326 -> [w342 w353]
              tunnel: w325 -> [_ w352]
              tunnel: [w342 w351] -> w324
              tunnel: w322 -> [_ w347]
              tunnel: [errorcluster {"status"=FALSE, "code"=0, "source"=""} ("error out") w346] -> w318
              tunnel: ["NI9205  (manual)" w345] -> w289
              frame True {
                n113 = Wait Until Next ms Multiple(millisecond multiple=u32 100 ("milliseconds to wait")) -> ()  [unwired: 1 out]
              }
              frame False {
                n114 = call-poly <vilib>:"DAQmx Read.vi"("task/channels in"=w353, "number of samples per channel"=20, "timeout"=1.0, "error in"=w352) -> ("task out"=w351:refnum<k21>, "data"=w348:dbl[][], "error out"=w346:errorcluster)  [unwired: 9 in]
                n115 = for {
                  N: w347 -> [_]
                  tunnel: w348 -> [w355] mode=indexing
                  tunnel: [w354] -> w345 mode=indexing
                  n116 = call-poly <vilib>:"Mean.vi"("X"=w355) -> ("mean"=w354:dbl)  [unwired: 1 out]
                }
              }
            }
            "NI9205" <- w289
            n117 = shared-variable "NI-cRIO-9049-020A5DED\\APC_SharedVars.lvlib\\PC_ControlSettings"() -> (w265:T1)  [unwired: 1 in, 1 out]
            "PC_ControlSettings" <- w265
            n118 = flat-sequence "MAIN SEQUENCE" {
              frame #0 {
                # "Digital input interface"
                # "AI_1 (consumer)"
                # "Sensor calibration (integrated in task)"
                # "Input variable mapping"
                # "NETWORK VARIABLES POLLING\n\n* Gets variables from other HW in the network\n* External requests"
                # "Analog input interface"
                # "INPUT INTERFACES"
              }
              frame #1 {
                # "subsystem modelling and diagnostics"
                # "subsystem modelling and diagnostics"
                # "subsystem modelling and diagnostics"
                # "subsystem modelling and diagnostics"
                # "subsystem modelling and diagnostics"
                # "Warnings and errors merging"
                # "supervisory control\n(decides subsystem, control mode and settings)"
                # "If MASTER"
              }
              frame #2 {
                # "subsystem controllers"
                # "subsystem controllers"
                # "subsystem controllers"
                # "subsystem controllers"
                # "subsystem controllers"
                # "subsystem controllers"
                # "subsystem controllers"
              }
              frame #3 {
                # "Digital output interface"
                # "Analog output interface"
                # "Output variable calibration"
                # "Output variable mapping"
                # "LOGGING (producer loop)"
                # "NETWORK  VARIABLES PUBLISH"
              }
            }
            n119 = call "APC_9056_9049SharedVarPolling.vi"("Number of signals"=w315) -> ("9049_CycleAveragedVariables"=w283:dbl[])  [unwired: 1 out]
            "9049_CycleAveragedVariables" <- w283
            n120 = call "APC_PID_VariableMapping.vi"("Index of array for 9056"=w284, "Index of array for 9049"=w285, "9049_CycleAveragedVariables"=w283) -> ("Output cluster"=w282:T8)  [unwired: 1 in, 2 out]
            n121 = call "APC_9056_WatchDog.vi"() -> ("MTRnotResponding"=→"MTRnotResponding":bool, "PCnotResponding"=w260:bool, "9049notResponding"=→"9049notResponding":bool, "9056notResponding"=w253:bool)  [unwired: 4 in]
            "9056notResponding" <- w253
            "PCnotResponding" <- w260
            n122 = call "APC_9056_MTRsignals.vi"("PC_ControlSettings"=w265) -> ("MTR signals array"=w266:dbl[])
            n123 = local read "AODODI_raster"() -> (w286:dbl[])
            n124 = shared-variable "NI-cRIO-9049-020A5DED\\APC_SharedVars.lvlib\\ForceState_SM"("ForceState") -> ()  [unwired: 1 in, 1 out]
            n125 = shared-variable "NI-cRIO-9049-020A5DED\\APC_SharedVars.lvlib\\ManualState_SM"("ManualState") -> ()  [unwired: 1 in, 1 out]
            n126 = local read "NI9208"() -> (w288:dbl[])
            n127 = local read "NI9214"() -> (w287:dbl[])
            n128 = flat-sequence {
              frame #0 {
                # "Gets queue"
              }
              frame #1 {
                # "Saves file(s)"
              }
            }
            n129 = flat-sequence {
              frame #0 {
                # "Sensor calibration (integrated in task)"
                # "AI_1"
              }
              frame #1 {
                # "Publish data for other loops"
              }
            }
            n130 = Or(x=w253, y=w260) -> (x .or. y?=w261:bool)
            n131 = Select(t=i8 -1 ("SYSTEM STATE"), s=w261, f=i8 3) -> (s? t:f=w257:i8)
            "s? t:f" <- w257
            n132 = Tick Count (ms)() -> (millisecond timer value=w292:u32)
            n133 = feedback #3(i8 0 ("SYSTEM STATE")) -> (w290:i8)
            "SYSTEM STATE" <- w290
            n134 = call "APC_9056_WarningIntegration.vi"("NI9205"=w289, "CURRENT SYSTEM STATE"=w290, "NI9208"=w288, "NI9214"=w287, "input cluster"=w282) -> ("STATE LIMITATION FROM WARNINGS"=w256:i8)  [unwired: 3 in]
            n135 = Max & Min(x=w257, y=w256) -> (min(x,y)=w255:i8)  [unwired: 1 out]
            n136 = call "APC_9056_StateMachine.vi"("ManualState"="ManualState", "ForceState"="ForceState", "PC_ControlSettings"=w265, "STATE LIMITATION FROM WARNINGS"=w255, "CURRENT SYSTEM STATE"=w290) -> ("SYSTEM STATE"=w263:i8)  [unwired: 4 in]
            n137 = Build Array (concatenate)(w292, w263, w289, w288, w287, w286, w266) -> (w314:dbl[])
            n138 = call "APC_9056_SharedVarBroadcast.vi"("9056_IOvector"=w314) -> ()
            n139 = call "APC_PID_VariableMapping.vi"("Index of array for 9056"=w284, "Index of array for 9049"=w285, "9056 IO"=w314, "9049_CycleAveragedVariables"=w283) -> ("Output cluster"=w310:T8)  [unwired: 2 out]
            n140 = Build Array (concatenate)(w314, w283) -> (w312:dbl[])
            n141 = Array Size(array=w312) -> (size(s)=→"size(s) 2":i32)
            n142 = feedback-in #3(w263) -> ()
            n143 = Unbundle By Name(w265) -> ("PID control references.NG"=w305:bool, "PID control references.Ar"=w304:bool, "PID control references.O2"=w303:bool, "PID control references.Intake vent"=w307:bool, "PID control references.Cross vent"=w308:bool, "PID control references.Exhaust vent"=w309:bool)
            n144 = call "APC_9056_O2Control.vi"("PC_ControlSettings"=w265, "input cluster"=w310) -> ("O2-FC-001-REF"=w299:dbl)  [unwired: 1 in]
            n145 = call "APC_9056_ArControl.vi"("input cluster"=w310) -> ("AR-PC-002-REF"=w298:dbl)  [unwired: 2 in]
            n146 = call "APC_9056_NGControl.vi"("PC_ControlSettings"=w265, "input cluster"=w310) -> ("NG-FC-001-REF"=w297:dbl)  [unwired: 1 in]
            n147 = call "APC_9056_TcoolantControl.vi"("PC_ControlSettings"=w265, "input cluster"=w310) -> ("EC-FC-001-REF"=w296:dbl)  [unwired: 1 in]
            n148 = call "APC_9056_TexhControl.vi"("input cluster"=w310) -> ("SW-FC-004-REF"=w295:dbl)  [unwired: 2 in]
            n149 = call "APC_9056_ToilControl.vi"("PC_ControlSettings"=w265, "input cluster"=w310) -> ("SW-FC-009-REF"=w294:dbl)  [unwired: 1 in]
            n150 = call "APC_9056_DynoControl.vi"("PC_ControlSettings"=w265, "input cluster"=w310) -> ("DYNO-REF"=w293:dbl)  [unwired: 1 in]
            n151 = shared-variable "NI-cRIO-9049-020A5DED\\APC_SharedVars.lvlib\\SystemState_SM"(w263) -> ()  [unwired: 1 in, 1 out]
            n152 = case shown="True" "Override controllers" {
              tunnel: w299 -> [w327 _]
              tunnel: w298 -> [w328 _]
              tunnel: w297 -> [w329 _]
              tunnel: w296 -> [w330 _]
              tunnel: w295 -> [w331 _]
              tunnel: w294 -> [w332 _]
              tunnel: w293 -> [w333 _]
              tunnel: [w333 "DYNO-REF"] -> w274
              tunnel: [w332 "SW-FC-009-REF"] -> w273
              tunnel: [w331 "SW-FC-004-REF"] -> w272
              tunnel: [w330 "EC-FC-001-REF"] -> w271
              tunnel: [w329 "NG-FC-001-REF"] -> w270
              tunnel: [w328 "AR-PC-002-REF"] -> w269
              tunnel: [w327 "O2-FC-001-REF"] -> w268
              frame False {
              }
              frame True {
              }
            }
            "SW-FC-004-REF" <- w272
            "NG-FC-001-REF" <- w270
            "EC-FC-001-REF" <- w271
            "SW-FC-009-REF" <- w273
            "O2-FC-001-REF" <- w268
            "AR-PC-002-REF" <- w269
            "DYNO-REF" <- w274
            n153 = shared-variable "NI-cRIO-9049-020A5DED\\APC_SharedVars.lvlib\\WarningLimits_SM"(w255) -> ()  [unwired: 1 in, 1 out]
            n154 = Enqueue Element(queue=w323, element=w312) -> ()  [unwired: 2 in, 3 out]
            n155 = Or(x=w318, y=FALSE ("Stop DAQ")) -> (x .or. y?=w316:bool)
            n156 = Not(x=w307) -> (.not. x?=w302:bool)
            n157 = Not(x=w308) -> (.not. x?=w301:bool)
            n158 = Not(x=w309) -> (.not. x?=w300:bool)
            n159 = case shown="False" "Override switchs from PC" {
              tunnel: w305 -> [_ w362]
              tunnel: w304 -> [_ w363]
              tunnel: w303 -> [_ w364]
              tunnel: w302 -> [_ w365]
              tunnel: w301 -> [_ w366]
              tunnel: w300 -> [_ w367]
              tunnel: ["ExhVent" w367] -> w275
              tunnel: ["CrossVent" w366] -> w276
              tunnel: ["IntVent" w365] -> w277
              tunnel: ["O2" w364] -> w278
              tunnel: ["Ar" w363] -> w279
              tunnel: ["NG" w362] -> w280
              frame True {
              }
              frame False {
              }
            }
            "NG-FV-001" <- w280
            "O2-PV-004" <- w279
            "AR-PV-004" <- w278
            "WF-FC-001" <- w277
            "WF-FC-002" <- w276
            "WF-FC-003" <- w275
            n160 = Tick Count (ms)() -> (millisecond timer value=w319:u32)
            n161 = feedback #4() -> (w320:u32)  [unwired: 1 in]
            n162 = feedback-in #4(w319) -> ()
            n163 = Subtract(x=w319, y=w320) -> (x-y=→"elapsed time 9205":u32)
            "NumChans_TEST" <- w322
            "task out_TEST" <- w326
            "error out TEST" <- w325
          }
          n164 = node-c288() -> ()  [unwired: 1 in, 1 out]
        }
        frame #1 {
          # "Let system think..."
          n165 = node-c288() -> ()  [unwired: 1 in, 1 out]
          n166 = call <vilib>:"DAQmx Stop Task.vi"("task/channels in"=w372, "error in"=w371) -> ("task out"=w370:refnum<k21>, "error out"=w369:errorcluster)  [unwired: 12 in]
          n167 = Wait Until Next ms Multiple(millisecond multiple=u32 1000 ("milliseconds to wait")) -> ()  [unwired: 1 out]
          n168 = node-c288() -> ()  [unwired: 1 in, 1 out]
        }
      }
    }
    n169 = node-c288(w229) -> ()
  }
  n170 = while {
    tunnel: w7 -> [w380]
    tunnel: "error in" -> [w386]
    tunnel: [w383] -> _
    tunnel: [w382] -> _
    stop <- FALSE ("Stop DAQ 5") stop-if-true
    n171 = property class="DAQmx Task"(reference=w380) -> ("NumChans"=w379:u32)  [unwired: 1 in, 2 out]
    n172 = call <vilib>:"DAQmx Start Task.vi"("task/channels in"=w380, "error in"=w386) -> ("task out"=w385:refnum<k21>, "error out"=w384:errorcluster)  [unwired: 12 in]
    n173 = node-c288(300 ("Priority")) -> (w389:T4)  [unwired: 3 in]
    n174 = timed-sequence {
      timing: w389 -> [_]
      timing-out: [_] -> w388
      tunnel: w385 -> [w396]
      tunnel: w384 -> [w395]
      tunnel: [w392] -> w383
      tunnel: [w391] -> w382
      tunnel: w379 -> [w390]
      n175 = timed-flat-sequence {
        tunnel: w396 -> [w401]
        tunnel: w395 -> [w400]
        tunnel: [w399] -> w394
        tunnel: [w398] -> w393
        tunnel: w390 -> [w397]
        tunnel: w394 -> [w435]
        tunnel: w393 -> [w434]
        tunnel: [w433] -> w392
        tunnel: [w432] -> w391
        frame #0 {
          n176 = node-c288() -> ()  [unwired: 1 in, 1 out]
          n177 = while {
            tunnel: w401 -> [w415]
            tunnel: w400 -> [w414]
            tunnel: [w413] -> w399
            tunnel: [w406] -> w398
            tunnel: w397 -> [w412]
            stop <- w407 stop-if-true
            # "AI3 - Thermocouple"
            n178 = case shown="False" "emulate 9214" {
              tunnel: w415 -> [w417 w428]
              tunnel: w414 -> [_ w427]
              tunnel: [w417 w426] -> w413
              tunnel: w412 -> [_ w422]
              tunnel: [errorcluster {"status"=FALSE, "code"=0, "source"=""} ("error out") w421] -> w406
              tunnel: ["NI9214  (manual)" w420] -> w405
              frame True {
                n179 = Wait Until Next ms Multiple(millisecond multiple=u32 100 ("milliseconds to wait")) -> ()  [unwired: 1 out]
              }
              frame False {
                n180 = call-poly <vilib>:"DAQmx Read.vi"("task/channels in"=w428, "number of samples per channel"=1, "timeout"=5.0, "error in"=w427) -> ("task out"=w426:refnum<k21>, "data"=w423:dbl[][], "error out"=w421:errorcluster)  [unwired: 9 in]
                n181 = for {
                  N: w422 -> [_]
                  tunnel: w423 -> [w430] mode=indexing
                  tunnel: [w429] -> w420 mode=indexing
                  n182 = call-poly <vilib>:"Mean.vi"("X"=w430) -> ("mean"=w429:dbl)  [unwired: 1 out]
                }
              }
            }
            "NI9214" <- w405
            n183 = Tick Count (ms)() -> (millisecond timer value=w409:u32)
            n184 = feedback #5() -> (w410:u32)  [unwired: 1 in]
            n185 = feedback-in #5(w409) -> ()
            n186 = Subtract(x=w409, y=w410) -> (x-y=→"elapsed time 9214":u32)
            n187 = Or(x=w406, y=FALSE ("Stop DAQ 6")) -> (x .or. y?=w407:bool)
          }
          n188 = node-c288() -> ()  [unwired: 1 in, 1 out]
        }
        frame #1 {
          # "Let system think..."
          n189 = node-c288() -> ()  [unwired: 1 in, 1 out]
          n190 = call <vilib>:"DAQmx Stop Task.vi"("task/channels in"=w435, "error in"=w434) -> ("task out"=w433:refnum<k21>, "error out"=w432:errorcluster)  [unwired: 12 in]
          n191 = Wait Until Next ms Multiple(millisecond multiple=u32 1000 ("milliseconds to wait")) -> ()  [unwired: 1 out]
          n192 = node-c288() -> ()  [unwired: 1 in, 1 out]
        }
      }
    }
    n193 = node-c288(w388) -> ()
  }
  n194 = while {
    tunnel: w8 -> [w442]
    tunnel: "error in" -> [w449]
    tunnel: [w446] -> _
    tunnel: [w445] -> _
    stop <- FALSE ("Stop DAQ 3") stop-if-true
    n195 = property class="DAQmx Task"(reference=w442) -> ("NumChans"=w443:u32)  [unwired: 1 in, 2 out]
    n196 = call <vilib>:"DAQmx Start Task.vi"("task/channels in"=w442, "error in"=w449) -> ("task out"=w448:refnum<k21>, "error out"=w447:errorcluster)  [unwired: 12 in]
    n197 = node-c288(300 ("Priority")) -> (w452:T4)  [unwired: 3 in]
    n198 = timed-sequence {
      timing: w452 -> [_]
      timing-out: [_] -> w451
      tunnel: w448 -> [w459]
      tunnel: w447 -> [w458]
      tunnel: [w455] -> w446
      tunnel: [w454] -> w445
      tunnel: w443 -> [w453]
      n199 = timed-flat-sequence {
        tunnel: w459 -> [w464]
        tunnel: w458 -> [w463]
        tunnel: [w462] -> w457
        tunnel: [w461] -> w456
        tunnel: w453 -> [w460]
        tunnel: w457 -> [w498]
        tunnel: w456 -> [w497]
        tunnel: [w496] -> w455
        tunnel: [w495] -> w454
        frame #0 {
          n200 = node-c288() -> ()  [unwired: 1 in, 1 out]
          n201 = while {
            tunnel: w464 -> [w478]
            tunnel: w463 -> [w477]
            tunnel: [w476] -> w462
            tunnel: [w469] -> w461
            tunnel: w460 -> [w475]
            stop <- w470 stop-if-true
            # "AI2 - Current"
            n202 = case shown="False" "emulate 9208" {
              tunnel: w478 -> [w480 w491]
              tunnel: w477 -> [_ w490]
              tunnel: [w480 w489] -> w476
              tunnel: w475 -> [_ w485]
              tunnel: [errorcluster {"status"=FALSE, "code"=0, "source"=""} ("error out") w484] -> w469
              tunnel: ["NI9208  (manual)" w483] -> w468
              frame True {
                n203 = Wait Until Next ms Multiple(millisecond multiple=u32 100 ("milliseconds to wait")) -> ()  [unwired: 1 out]
              }
              frame False {
                n204 = call-poly <vilib>:"DAQmx Read.vi"("task/channels in"=w491, "number of samples per channel"=1, "timeout"=5.0, "error in"=w490) -> ("task out"=w489:refnum<k21>, "data"=w486:dbl[][], "error out"=w484:errorcluster)  [unwired: 9 in]
                n205 = for {
                  N: w485 -> [_]
                  tunnel: w486 -> [w493] mode=indexing
                  tunnel: [w492] -> w483 mode=indexing
                  n206 = call-poly <vilib>:"Mean.vi"("X"=w493) -> ("mean"=w492:dbl)  [unwired: 1 out]
                }
              }
            }
            "NI9208" <- w468
            n207 = Tick Count (ms)() -> (millisecond timer value=w472:u32)
            n208 = feedback #6() -> (w473:u32)  [unwired: 1 in]
            n209 = feedback-in #6(w472) -> ()
            n210 = Subtract(x=w472, y=w473) -> (x-y=→"elapsed time 9208":u32)
            n211 = Or(x=w469, y=FALSE ("Stop DAQ 4")) -> (x .or. y?=w470:bool)
          }
          n212 = node-c288() -> ()  [unwired: 1 in, 1 out]
        }
        frame #1 {
          # "Let system think..."
          n213 = node-c288() -> ()  [unwired: 1 in, 1 out]
          n214 = call <vilib>:"DAQmx Stop Task.vi"("task/channels in"=w498, "error in"=w497) -> ("task out"=w496:refnum<k21>, "error out"=w495:errorcluster)  [unwired: 12 in]
          n215 = node-c288() -> ()  [unwired: 1 in, 1 out]
          n216 = Wait Until Next ms Multiple(millisecond multiple=u32 1000 ("milliseconds to wait")) -> ()  [unwired: 1 out]
        }
      }
    }
    n217 = node-c288(w451) -> ()
  }
